vi "PicoScope4000ExampleRapidBlockBulk.vi"() -> ()   [LabVIEW 2012]
doc: "This example demonstrates how to use the PicoScope Labview library to collect data using rapid block mode, retrieving the data values in bulk."
uses:
  shared/PicoBuffers.ctl
  shared/Segment Range.ctl
  shared/Acquisition Settings.ctl
  shared/nSegments.ctl
  PicoScope4000Lib/PicoScope4000AnalogChannelSettingsIEPE.ctl
  PicoScope4000Lib/PicoScope4000Buffer and Transfer Settings.ctl
panel:
  in  "Channel B Settings":T1={"Enabled"=FALSE, "Range"=6, "Bandwidth Limit"=0, "Coupling"=1} {"Coupling" items=["AC", "DC", "IEPE"]; "Bandwidth Limit" items=["Off", "200kHz"]; "Range" items=["10 mV", "20 mV", "50 mV", "100 mV", "200 mV", "500 mV", "1 V", "2 V", "5 V", "10 V", "20 V", "50 V ", "100 V"]}
  out "Overflow":i16[](array[numeric]) format="%04b"
  in  "Trigger Settings":T2={"Trigger Enabled"=FALSE, "Trigger Source"=enum."Channel A", "Trigger Threshold (Volts)"=0.0, "Trigger Direction"=2, "Trigger Delay (samples)"=0, "Auto Trigger Time (ms)"=1000} {"Trigger Direction" items=["Rising"=2, "Falling"=3]}
  out "nCaptures":u64 format="%.4p"
  in  "Channel A Settings":T1={"Enabled"=TRUE, "Range"=6, "Bandwidth Limit"=0, "Coupling"=1} {"Coupling" items=["AC", "DC", "IEPE"]; "Bandwidth Limit" items=["Off", "200kHz"]; "Range" items=["10 mV", "20 mV", "50 mV", "100 mV", "200 mV", "500 mV", "1 V", "2 V", "5 V", "10 V", "20 V", "50 V ", "100 V"]}
  in  "PicoScope 4262 Ext. Trigger Range":u32(ring)=5 items=["500 mV"=5, "5 V"=8]
  out "Unit Info":T3
  in  "Stop Display":bool
  out "Capture Complete":bool
  in  "Run":bool
  in  "Display Buffer Index":i32
  in  "Segment Range":T4={"fromSegmentIndex"=0, "toSegmentIndex"=9} {"toSegmentIndex" format="%.4p"; "fromSegmentIndex" format="%.4p"}
  in  "nSegments":T5=10 format="%.4p"
  out "error out":errorcluster
  in  "Data file":path=path "PicoScope4000ExampleRapidBlock ChA Data"
  in  "Buffer and Transfer Settings":T6={"startIndex"=0, "Samples"=1000000, "Down Sample Ratio"=1, "Down-Sample Mode"=0} {"Down-Sample Mode" items=["None", "Aggregate", "Average"]; "Down Sample Ratio" step=1; "Samples" format="%_6p"}
  in  "Acquisition Settings":T7={"preTriggerSamples"=0, "postTriggerSamples"=1000000, "timebase"=5} {"postTriggerSamples" format="%_6p"; "preTriggerSamples" format="%_6p"}
  out "Properties Panel":T8 {"Max Total Capture Time Available (sec)" format="%.3p"; "Sample Frequency" format="%.6p"; "Sample Rate" format="%.3p"; "Max Samples Available" format="%_6p"; "Total Capture Time (sec)" format="%.3p"}
  in  "stop":bool
  out "Analog Channels":cluster{i32, dbl, "Data":dbl[]}[](graph)
  in  "Serial Number":string
  in  "Use Serial Number":bool
  in  "error in (no error)":errorcluster
  # "Number of\nSegments to Capture"
  # "Bit 0 = ChA"
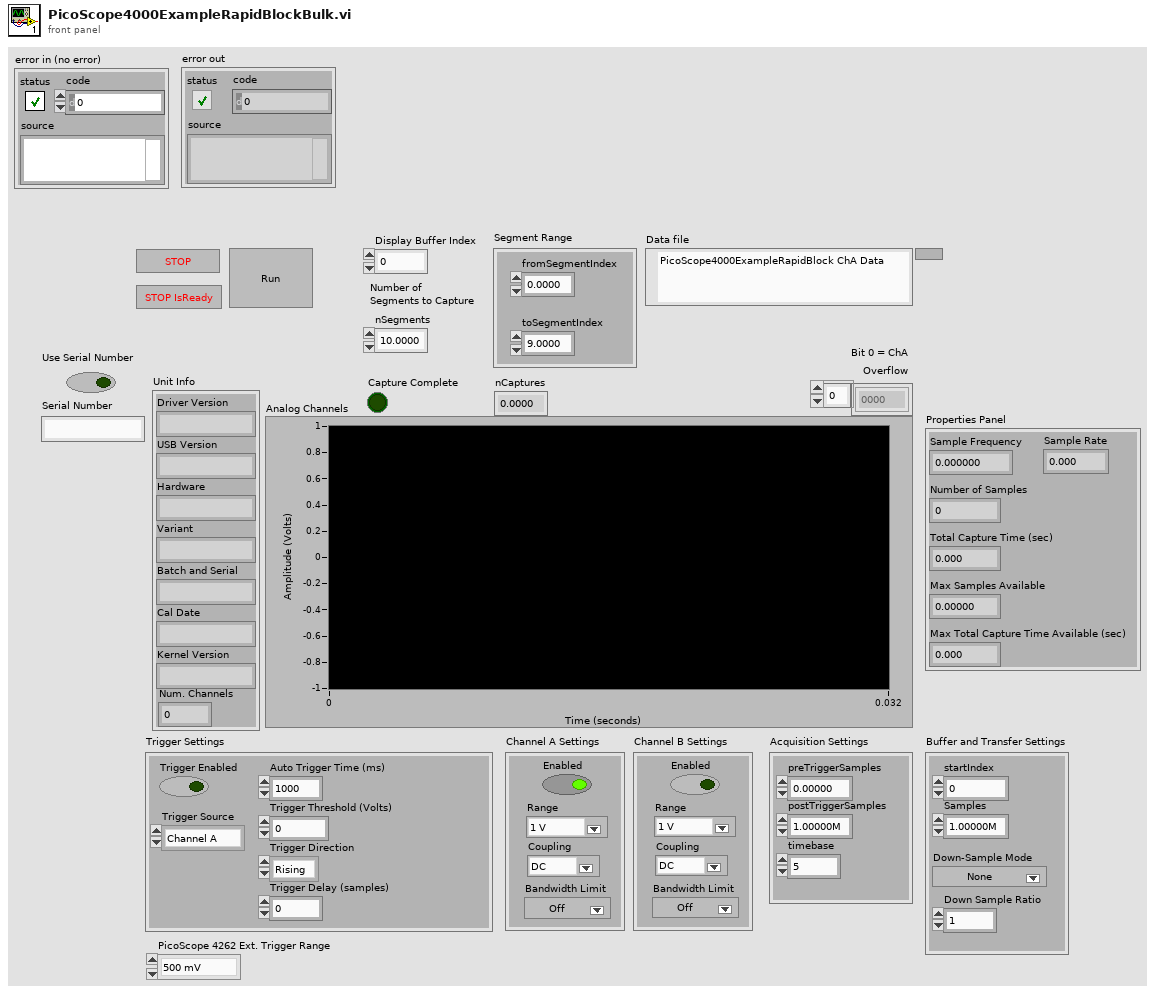
[diagram p1: front panel]
types:
  T1 = typedef "PicoScope4000AnalogChannelSettingsIEPE.ctl" = cluster{"Enabled":bool, "Range":u16, "Bandwidth Limit":i16, "Coupling":u16}
  T2 = cluster{"Trigger Enabled":bool, "Trigger Source":enum16{"Channel A", "Channel B", "Channel C", "Channel D", "Channel E", "Channel F", "Channel G", "Channel H"}, "Trigger Threshold (Volts)":dbl, "Trigger Direction":u16, "Trigger Delay (samples)":u32, "Auto Trigger Time (ms)":i16}
  T3 = cluster{"Driver Version":string, "USB Version":string, "Hardware":string, "Variant":string, "Batch and Serial":string, "Cal Date":string, "Kernel Version":string, "Num. Channels":i16}
  T4 = typedef "Segment Range.ctl" = cluster{"fromSegmentIndex":u64, "toSegmentIndex":u64}
  T5 = typedef "nSegments.ctl" = u64
  T6 = typedef "PicoScope4000Buffer and Transfer Settings.ctl" = cluster{"startIndex":u64, "Samples":u64, "Down Sample Ratio":u64, "Down-Sample Mode":u32}
  T7 = typedef "Acquisition Settings.ctl" = cluster{"preTriggerSamples":u64, "postTriggerSamples":u64, "timebase":u32}
  T8 = cluster{"Sample Frequency":dbl, "Sample Rate":dbl, "Max Samples Available":u64, "Number of Samples":u64, "Total Capture Time (sec) ":dbl, "Max Total Capture Time Available (sec)":dbl}
  T9 = enum16{"open", "open or create", "create or replace", "create", "open (read-only)"}
  T10 = typedef "PicoBuffers.ctl" = cluster{"Max Buffer Pointers":u64[][][], "Min Buffer Pointers":u64[][][], "StreamingDataInfo":cluster{"Channel":u32, "Down-Sample Mode":u32, "PICO_DATA_TYPE":enum32{"PICO_INT8_T", "PICO_INT16_T", "PICO_INT32_T", "PICO_UINT32_T", "PICO_INT64_T", ""}, "Samples":i32, "bufferIndex":u64, "startIndex":i32, "overflow":i16}[][]}
  T11 = cluster{"Channel A Buffer":i16[], "Channel B Buffer":i16[], "Channel C Buffer":i16[], "Channel D Buffer":i16[], "Channel E Buffer":i16[], "Channel F Buffer":i16[], "Channel G Buffer":i16[], "Channel H Buffer":i16[], "Port 0 Buffer":i16[], "Port 1 Buffer":i16[]}[]
  T12 = cluster{"Channel A Buffer":i16[], "Channel B Buffer":i16[], "Channel C Buffer":i16[], "Channel D Buffer":i16[], "Channel E Buffer":i16[], "Channel F Buffer":i16[], "Channel G Buffer":i16[], "Channel H Buffer":i16[], "Port 0 Buffer":i16[], "Port 1 Buffer":i16[]}
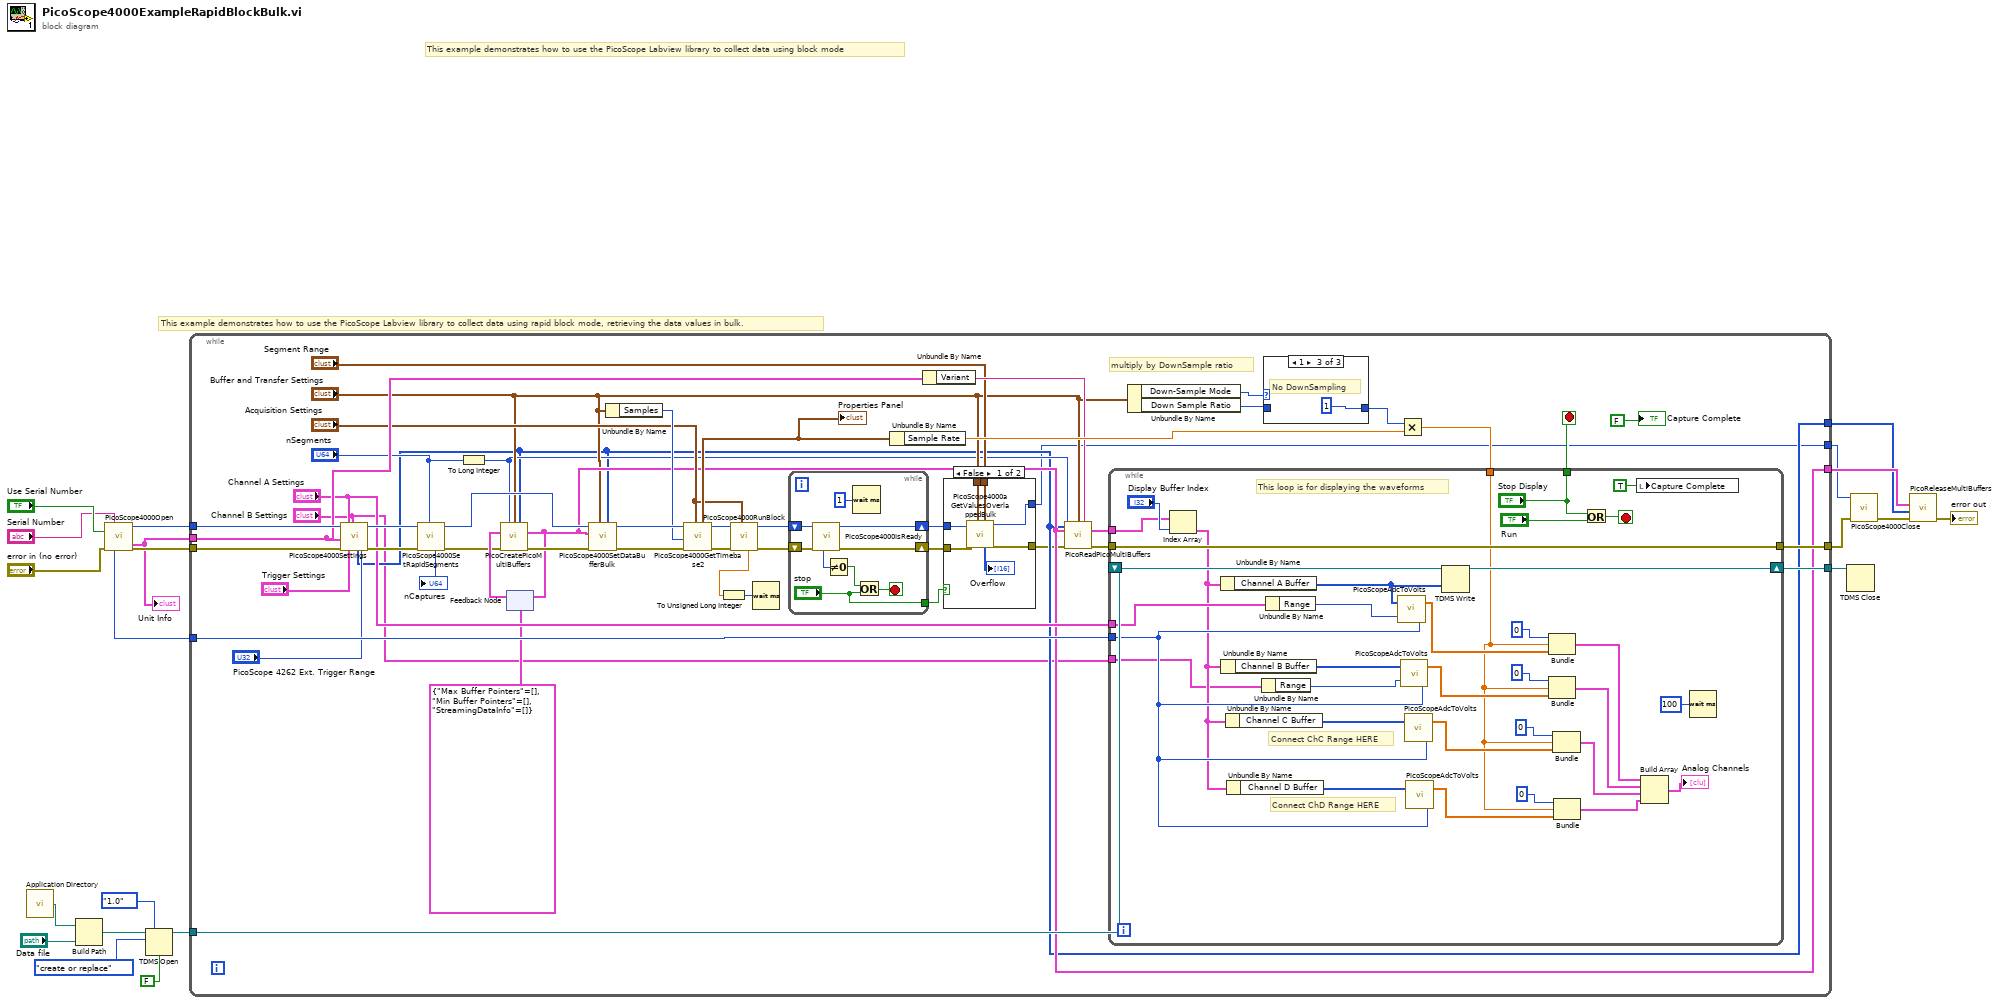
[diagram p0: block diagram]
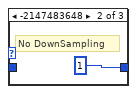
[diagram p4: hidden frame]
diagram:
  # "This example demonstrates how to use the PicoScope Labview library to collect data using rapid block mode, retrieving the data values in bulk."
  # "This example demonstrates how to use the PicoScope Labview library to collect data using block mode"
  n1 = call <vilib>:"Application Directory.vi"() -> ("Application Directory"=w14:path)
  n2 = Build Path(base path=w14, name or relative path="Data file") -> (appended path=w15:path)
  n3 = call "PicoScope4000Open.vi"("Serial Number"="Serial Number", "Use Serial Number"="Use Serial Number", "error in (no error)"="error in (no error)") -> ("handle"=w10:i16, "Max ADC value"=w11:i16, "Unit Info"=w5:T3, "error out"=w6:errorcluster)  [unwired: 9 in]
  "Unit Info" <- w5
  n4 = TDMS Open(6:FALSE ("disable buffering? (T)"), 7:enum16{"1.0", "2.0"}."1.0" ("file format version (2.0)"), 10:T9."create or replace" ("operation (0:open)"), 11:w15) -> (3:w12:refnum<k34>)  [unwired: 2 in, 1 out]
  n5 = while {
    tunnel: w11 -> [w55]
    tunnel: [w26] -> w20
    tunnel: [w28] -> w2
    tunnel: [w32] -> w21
    tunnel: [w70] -> w13
    tunnel: w12 -> [w69]
    tunnel: w10 -> [w57]
    tunnel: [w56] -> w4
    tunnel: w6 -> [w50]
    tunnel: w5 -> [w46]
    stop <- w59 stop-if-true
    # "multiply by DownSample ratio"
    n6 = call "PicoScope4000Settings.vi"("handle in"=w57, "Unit Info"=w46, "error in"=w50, "Channel A Settings"="Channel A Settings", "Trigger Settings"="Trigger Settings", "Channel B Settings"="Channel B Settings", "PicoScope 4262 Ext. Trigger Range"="PicoScope 4262 Ext. Trigger Range") -> ("Enabled array"=w28:i16[], "handle out"=w49:i16, "error out"=w48:errorcluster)  [unwired: 10 in]
    n7 = call "PicoScope4000SetRapidSegments.vi"("nSegments"="nSegments", "error in (no error)"=w48, "handle in"=w49) -> ("error out"=w68:errorcluster, "handle out"=w67:i16, "nCaptures"=→"nCaptures":u64)  [unwired: 6 in]
    n8 = To Long Integer(number="nSegments") -> (32bit integer=w30:i32)
    n9 = feedback #1(T10 {"Max Buffer Pointers"=[], "Min Buffer Pointers"=[], "StreamingDataInfo"=[]} ("Data Pointers")) -> (w72:T10)
    n10 = call "PicoCreatePicoMultiBuffers.vi"("Number of Buffers"=w30, "Buffer and Transfer Settings"="Buffer and Transfer Settings", "enabled array"=w28, "Data Pointers In"=w72, "error in (no error)"=w68) -> ("Data Pointers"=w32:T10, "error out"=w71:errorcluster)  [unwired: 9 in]
    n11 = feedback-in #1(w32) -> ()
    n12 = call "PicoScope4000SetDataBufferBulk.vi"("enabled array"=w28, "Buffer and Transfer Settings"="Buffer and Transfer Settings", "error in (no error)"=w71, "Data Pointers In"=w32, "handle in"=w67) -> ("error out"=w42:errorcluster, "handle out"=w41:i16)  [unwired: 5 in]
    n13 = Unbundle By Name("Buffer and Transfer Settings") -> ("Samples"=w40:u64)
    n14 = call "PicoScope4000GetTimebase2.vi"("Number of Samples"=w40, "Acquisition Settings"="Acquisition Settings", "error in (no error)"=w42, "handle in"=w41) -> ("error out"=w51:errorcluster, "handle out"=w52:i16, "Properties Panel"=w63:T8)  [unwired: 5 in]
    "Properties Panel" <- w63
    n15 = call "PicoScope4000RunBlock.vi"("Acquisition Settings"="Acquisition Settings", "error in (no error)"=w51, "handle in"=w52) -> ("error out"=w35:errorcluster, "handle out"=w36:i16, "timeIndisposedMs"=w24:dbl)  [unwired: 5 in, 1 out]
    n16 = To Unsigned Long Integer(number=w24) -> (unsigned 32bit integer=w25:u32)
    n17 = Wait (ms)(milliseconds to wait=w25) -> ()  [unwired: 1 out]
    n18 = while {
      shift-right: [w123] -> w33
      shift-left: w35 -> [w124]
      shift-right: [w122] -> w34
      shift-left: w36 -> [w121]
      tunnel: ["stop"] -> w23
      stop <- w118 stop-if-true
      n19 = call "PicoScope4000IsReady.vi"("error in (no error)"=w124, "handle in"=w121) -> ("error out"=w123:errorcluster, "handle out"=w122:i16, "ready"=w120:i16)  [unwired: 7 in]
      n20 = Not Equal To 0?(x=w120) -> (x != 0?=w119:bool)
      n21 = Wait (ms)(milliseconds to wait=u32 1) -> ()  [unwired: 1 out]
      n22 = Or(x=w119, y="stop") -> (x .or. y?=w118:bool)
    }
    n23 = Unbundle By Name(w63) -> ("Sample Rate"=w54:dbl)
    n24 = Unbundle By Name(w46) -> ("Variant"=w53:string)
    n25 = case shown="False" w23 {
      tunnel: "Segment Range" -> [w79 _]
      tunnel: w34 -> [w78 w81]
      tunnel: w33 -> [w77 w80]
      tunnel: "Buffer and Transfer Settings" -> [w76 _]
      tunnel: [w75 w80] -> w27
      tunnel: [w74 w81] -> w26
      frame False {
        n26 = call "PicoScope4000aGetValuesOverlappedBulk.vi"("Segment Range"=w79, "Buffer and Transfer Settings"=w76, "error in (no error)"=w77, "handle in"=w78) -> ("error out"=w75:errorcluster, "handle out"=w74:i16, "overflow"=→"Overflow":i16[])  [unwired: 4 in, 1 out]
      }
      frame True {
      }
    }
    n27 = call "PicoReadPicoMultiBuffers.vi"("enabled array"=w28, "Buffer and Transfer Settings"="Buffer and Transfer Settings", "Variant"=w53, "Data Pointers"=w32, "No of Buffers"=w30, "error in (no error)"=w27) -> ("MultiBuffers (Max or non-aggregated)"=w66:T11, "error out"=w60:errorcluster)  [unwired: 7 in, 1 out]
    n28 = Unbundle By Name("Buffer and Transfer Settings") -> ("Down-Sample Mode"=w64:u32, "Down Sample Ratio"=w65:u64)
    n29 = case shown="1" w64 {
      tunnel: [w125 u64 1 ("Down Sample Ratio") u64 1 ("Down Sample Ratio")] -> w61
      tunnel: w65 -> [w125 _ _]
      frame Default {
      }
      frame -2147483648 {
        # "No DownSampling"
      }
      frame 1 {
        # "No DownSampling"
      }
    }
    n30 = Multiply(x=w61, y=w54) -> (x*y=w62:dbl)
    n31 = while {
      tunnel: w55 -> [w85]
      tunnel: "Channel A Settings" -> [w115]
      tunnel: w66 -> [w95]
      tunnel: w62 -> [w87]
      shift-right: [w114] -> w70
      shift-left: w69 -> [w113]
      tunnel: [w101] -> w56
      tunnel: w60 -> [w101]
      tunnel: ["Stop Display"] -> w59
      tunnel: "Channel B Settings" -> [w82]
      stop <- w98 stop-if-true
      # "This loop is for displaying the waveforms"
      # "Connect ChD Range HERE"
      # "Connect ChC Range HERE"
      n32 = Index Array(array=w95, index="Display Buffer Index") -> (element=w84:T12)
      n33 = Unbundle By Name(w84) -> ("Channel A Buffer"=w103:i16[])
      n34 = Unbundle By Name(w84) -> ("Channel B Buffer"=w109:i16[])
      n35 = Unbundle By Name(w84) -> ("Channel C Buffer"=w93:i16[])
      n36 = Unbundle By Name(w84) -> ("Channel D Buffer"=w89:i16[])
      n37 = Unbundle By Name(w82) -> ("Range"=w83:u16)
      n38 = Unbundle By Name(w115) -> ("Range"=w111:u16)
      n39 = call "PicoScopeAdcToVolts.vi"("Max_adc"=w85, "Range Index"=w111, "Data"=w103) -> ("Data"=w104:dbl[])
      n40 = call "PicoScopeAdcToVolts.vi"("Max_adc"=w85, "Range Index"=w83, "Data"=w109) -> ("Data"=w108:dbl[])
      n41 = call "PicoScopeAdcToVolts.vi"("Max_adc"=w85, "Data"=w93) -> ("Data"=w92:dbl[])  [unwired: 1 in]
      n42 = call "PicoScopeAdcToVolts.vi"("Max_adc"=w85, "Data"=w89) -> ("Data"=w88:dbl[])  [unwired: 1 in]
      n43 = TDMS Write(0:w113, 9:w103) -> (4:w114:refnum<k34>)  [unwired: 4 in, 3 out]
      n44 = Bundle(0, w87, "Data"=w104) -> (w107:cluster{i32, dbl, "Data":dbl[]})  [unwired: 1 in]
      n45 = Bundle(0, w87, "Data"=w108) -> (w106:cluster{i32, dbl, "Data":dbl[]})  [unwired: 1 in]
      n46 = Bundle(0, w87, "Data"=w92) -> (w91:cluster{i32, dbl, "Data":dbl[]})  [unwired: 1 in]
      n47 = Bundle(0, w87, "Data"=w88) -> (w86:cluster{i32, dbl, "Data":dbl[]})  [unwired: 1 in]
      n48 = Or(x="Stop Display", y="Run") -> (x .or. y?=w98:bool)
      n49 = local write "Capture Complete"(TRUE ("Capture Complete")) -> ()
      n50 = Build Array(w107, w106, w91, w86) -> (→"Analog Channels":cluster{i32, dbl, "Data":dbl[]}[])
      n51 = Wait (ms)(milliseconds to wait=u32 100) -> ()  [unwired: 1 out]
    }
    "Capture Complete" <- FALSE ("Capture Complete")
  }
  n52 = TDMS Close(11:w13) -> ()  [unwired: 1 in, 2 out]
  n53 = call "PicoScope4000Close.vi"("error in (no error)"=w4, "handle"=w20) -> ("error out"=w3:errorcluster)  [unwired: 9 in]
  n54 = call "PicoReleaseMultiBuffers.vi"("error in (no error)"=w3, "Enabled array"=w2, "Data Pointers"=w21) -> ("error out"=→"error out":errorcluster)  [unwired: 8 in]
